vi "Check Data.vi"(7 "reset":bool, 10 "Input valid":bool=TRUE, 11 "IQ Stream":u64) -> (3 "errors":u32)   [LabVIEW 2016, in "Aurora Stream (NI 6592R) (FPGA).lvlib"]
uses:
  Aurora Stream (NI 6592R) (FPGA).lvlib
  <instrlib>/_niInstr/Basic Elements/v1/FPGA/Private/Count Up U32.vi
  <instrlib>/_niInstr/Basic Elements/v1/FPGA/niInstr Basic Elements v1 FPGA.lvlib
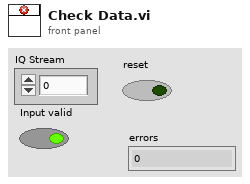
[diagram p1: front panel]
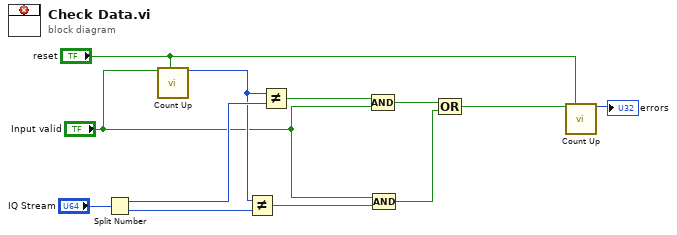
[diagram p0: block diagram]
diagram:
  n1 = Split Number(x="IQ Stream") -> (hi(x)=w12:u32, lo(x)=w9:u32)
  n2 = call-poly <instrlib>:"Count Up.vi"("increment"="Input valid", "reset"="reset") -> ("count out"=w7:u32)  [unwired: 13 in]
  n3 = Not Equal?(x=w7, y=w9) -> (x != y?=w5:bool)
  n4 = Not Equal?(x=w7, y=w12) -> (x != y?=w6:bool)
  n5 = Compound Arithmetic op=AND(w6, "Input valid") -> (w3:bool)
  n6 = Compound Arithmetic op=AND("Input valid", w5) -> (w2:bool)
  n7 = Compound Arithmetic op=OR(w3, w2) -> (w1:bool)
  n8 = call-poly <instrlib>:"Count Up.vi"("increment"=w1, "reset"="reset") -> ("count out"=→"errors":u32)  [unwired: 13 in]
